vi "SetupDefault.vi"(8 "error in (no error)":errorcluster, 10 "Alias":string, 11 "PwrMtr_RSNRPZ in":refnum<class "PwrMtr_RSNRPZ.lvclass">) -> (0 "error out":errorcluster, 3 "PwrMtr_RSNRPZ out":refnum<class "PwrMtr_RSNRPZ.lvclass">)   [LabVIEW 2014, in "PwrMtr_RSNRPZ.lvclass"]
uses:
  PwrMtr_RSNRPZ.lvclass
  PwrMtr_RSNRPZ.lvclass/PwrMtr_RSNRPZ.ctl
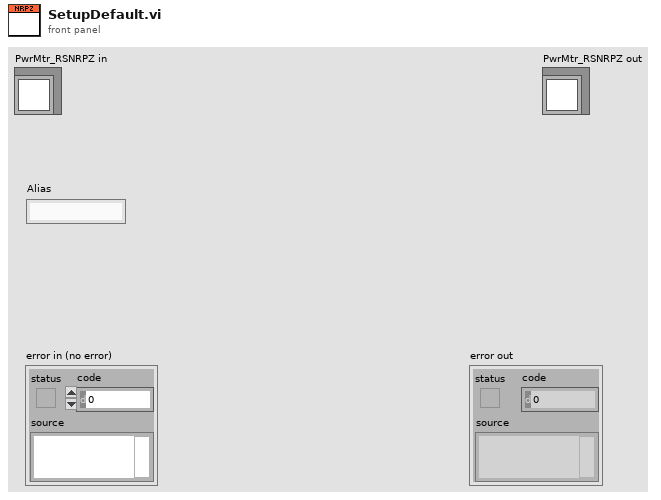
[diagram p1: front panel]
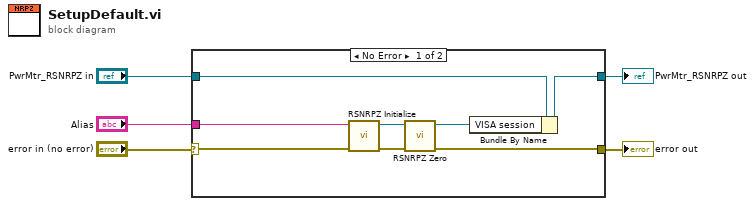
[diagram p0: block diagram]
diagram:
  n1 = case shown="No Error" "error in (no error)" {
    selector: "error in (no error)" -> [w11 w14]
    tunnel: "PwrMtr_RSNRPZ in" -> [w13 w15]
    tunnel: [w12 w15] -> w2
    tunnel: [w6 w14] -> w5
    tunnel: "Alias" -> [w10 _]
    frame No Error {
      n2 = call "RSNRPZ Initialize.vi"("error in (no error)"=w11, "Resource Name (USB::0x0aad::0x000b::100000)"=w10) -> ("error out"=w8:errorcluster, "dup VISA session"=w9:refnum<visa-resource-name>)  [unwired: 8 in]
      n3 = call "RSNRPZ Zero.vi"("error in (no error)"=w8, "VISA session"=w9) -> ("error out"=w6:errorcluster, "dup VISA session"=w7:refnum<visa-resource-name>)  [unwired: 8 in]
      n4 = Bundle By Name(cluster=w13, "VISA session"=w7) -> (w12:refnum<class "PwrMtr_RSNRPZ.lvclass">)
    }
    frame Error {
    }
  }
  "error out" <- w5
  "PwrMtr_RSNRPZ out" <- w2
